vi "方框循环运动子vi.vi"(5 "比例(um/步)":dbl=91.48, 6 "运行步数/um":dbl=2.0, 7 "error in (no error)":errorcluster, 8 "Device Address In":i32, 9 "DeviceKey In":string, 10 "Motor":i32, 11 "CmdLib In":refnum<k24>) -> (0 "error out":errorcluster, 1 "DeviceKey Out":string, 2 "Device Address Out":i32, 3 "CmdLib Out":refnum<k24>)   [LabVIEW 2018]
uses:
  CmdLib.dll
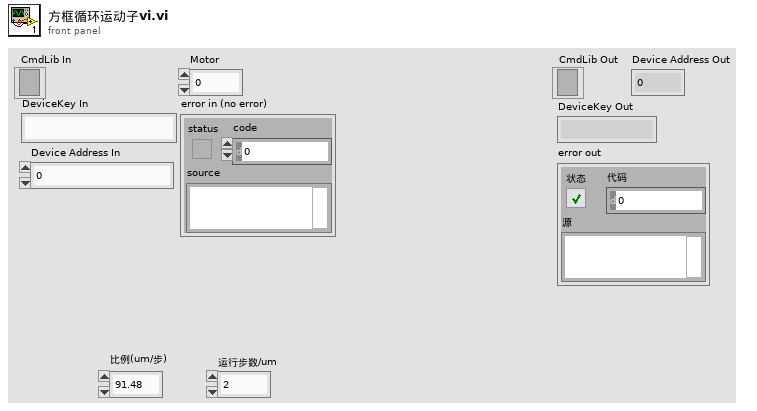
[diagram p1: front panel]
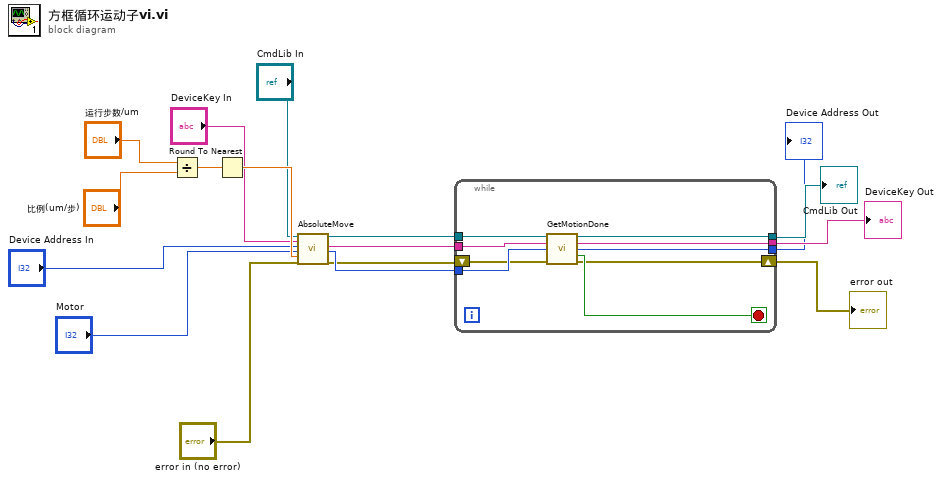
[diagram p0: block diagram]
diagram:
  n1 = Divide(x="运行步数/um", y="比例(um/步)") -> (x/y=w11:dbl)
  n2 = Round To Nearest(number=w11) -> (nearest integer value=w10:dbl)
  n3 = call "AbsoluteMove.vi"("CmdLib In"="CmdLib In", "DeviceKey In"="DeviceKey In", "Device Address In"="Device Address In", "Motor"="Motor", "Target Pos"=w10, "error in (no error)"="error in (no error)") -> ("CmdLib Out"=w17:refnum<k24>, "DeviceKey Out"=w16:string, "Device Address Out"=w15:i32, "error out"=w14:errorcluster)  [unwired: 10 in]
  n4 = while {
    tunnel: w17 -> [w26]
    tunnel: w16 -> [w25]
    tunnel: w15 -> [w24]
    shift-right: [w21] -> w1
    shift-left: w14 -> [w23]
    tunnel: [w20] -> w4
    tunnel: [w19] -> w3
    tunnel: [w18] -> w2
    stop <- w22 stop-if-true
    n5 = call "GetMotionDone.vi"("CmdLib In"=w26, "DeviceKey In"=w25, "Device Address In"=w24, "error in (no error)"=w23) -> ("CmdLib Out"=w20:refnum<k24>, "DeviceKey Out"=w19:string, "Device Address Out"=w18:i32, "Is Motion Done"=w22:bool, "error out"=w21:errorcluster)  [unwired: 7 in]
  }
  "CmdLib Out" <- w4
  "DeviceKey Out" <- w3
  "Device Address Out" <- w2
  "error out" <- w1
